vi "Insert New STDF File.vi"(8 "error in (no error)":errorcluster, 9 "STDF Files Per Tester":path[](array[path]), 10 "Tester #":u8, 11 "STDF File Parser in":refnum<class "STDF File Parser.lvclass">) -> (0 "error out":errorcluster, 3 "STDF File Parser out":refnum<class "STDF File Parser.lvclass">)   [LabVIEW 2018, in "STDF File Parser.lvclass"]
uses:
  STDF File Parser.lvclass
  STDF File Parser.lvclass/STDF File Parser.ctl
  <vilib>/Utility/error.llb/Error Cluster From Error Code.vi
  <vilib>/ErrorRing/Error Ring.xnode
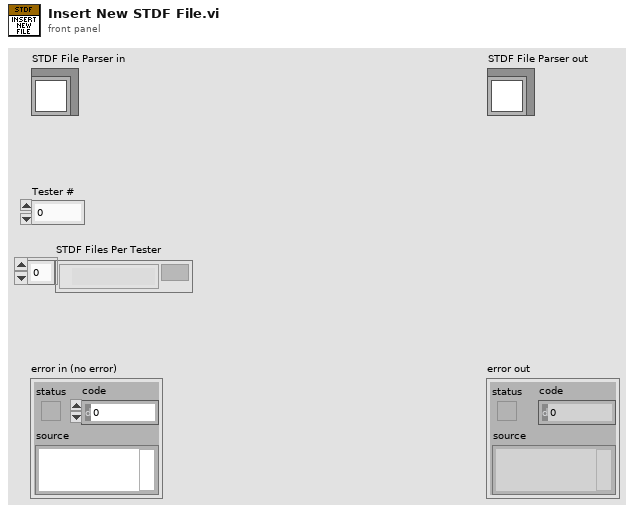
[diagram p1: front panel]
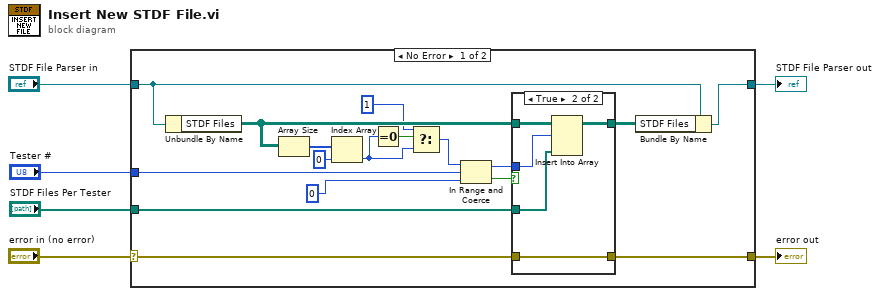
[diagram p0: block diagram]
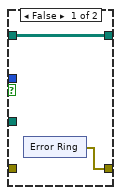
[diagram p2: hidden frame]
diagram:
  n1 = case shown="No Error" "error in (no error)" {
    selector: "error in (no error)" -> [w19 w36]
    tunnel: [w18 w36] -> w5
    tunnel: [w21 w37] -> w3
    tunnel: "STDF File Parser in" -> [w23 w37]
    tunnel: "Tester #" -> [w13 _]
    tunnel: "STDF Files Per Tester" -> [w11 _]
    frame No Error {
      n2 = Unbundle By Name(w23) -> ("STDF Files"=w20:path[][])
      n3 = Array Size(array=w20) -> (size(s)=w15:i32[])
      n4 = Index Array(array=w15, index=0) -> (element=w9:i32)
      n5 = Equal To 0?(x=w9) -> (x = 0?=w10:bool)
      n6 = Select(t=1, s=w10, f=w9) -> (s? t:f=w8:i32)
      n7 = In Range and Coerce(upper limit=w8, x=w13, lower limit=0) -> (coerced(x)=w17:i32, In Range?=w12:bool)
      n8 = case shown="True" w12 {
        tunnel: [w25 w35] -> w22
        tunnel: w20 -> [w25 w34]
        tunnel: w19 -> [_ w33]
        tunnel: [w24 w33] -> w18
        tunnel: w17 -> [_ w32]
        tunnel: w11 -> [_ w31]
        frame False {
          n9 = xnode "Error Ring"() -> ("error out"=w24:errorcluster)
        }
        frame True {
          n10 = Insert Into Array(array=w34, index (row)=w32, new element=w31) -> (w35:path[][])  [unwired: 1 in]
        }
      }
      n11 = Bundle By Name(cluster=w23, "STDF Files"=w22) -> (w21:refnum<class "STDF File Parser.lvclass">)
    }
    frame Error {
    }
  }
  "error out" <- w5
  "STDF File Parser out" <- w3
